vi "Read Info.vi"(8 "error in (no error)":errorcluster, 11 "OpenHW in":refnum<class "OpenHW.lvclass">) -> (0 "error out":errorcluster, 3 "OpenHW out":refnum<class "OpenHW.lvclass">)   [LabVIEW 2022 SP3, in "open-hw-mon-lv.lvlib" / "OpenHW.lvclass"]
uses:
  OpenHW.lvclass
  OpenHW.lvclass/OpenHW.ctl
  <vilib>/httpClient/LabVIEWHTTPClient.lvlib
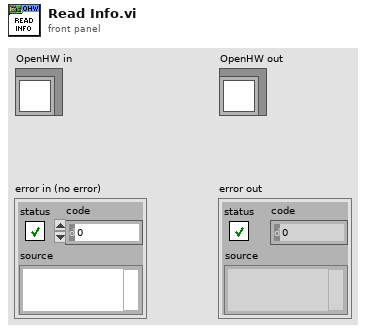
[diagram p1: front panel]
types:
  T1 = typedef "open-hw-mon-lv.lvlib/OpenHW.lvclass/HW Node.ctl" = cluster{"id":i32, "Text":string, "Value":string, "Min":string, "Max":string, "Parent":i32, "Children":i32[], "ImageURL":string}
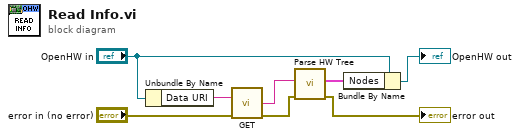
[diagram p0: block diagram]
diagram:
  n1 = Unbundle By Name("OpenHW in") -> ("Data URI"=w8:string)
  n2 = call <vilib>:"GET.vi"("url"=w8, "error in (no error)"="error in (no error)") -> ("body"=w7:string, "error out"=w5:errorcluster)  [unwired: 10 in, 2 out]
  n3 = call "Parse HW Tree.vi"("error in (no error)"=w5, "JSON"=w7) -> ("error out"=→"error out":errorcluster, "Nodes"=w2:T1[])  [unwired: 8 in]
  n4 = Bundle By Name(cluster="OpenHW in", "Nodes"=w2) -> (→"OpenHW out":refnum<class "OpenHW.lvclass">)
